vi "Main.vi"() -> ()   [LabVIEW 2021]
uses:
  Bronkhorst M13 Flow Meter/Settings Cluster.ctl
  Bronkhorst M13 Flow Meter/Bronkhorst M13 Flow Meter.lvlib
panel:
  in  "stop":bool
  in  "Bronkhorst Settings in":T1={"VISA resource name"="", "Simulated?"=FALSE, "Smoothing Steps"=1} {"Smoothing Steps" min=1 step=1}
  out "error out":errorcluster
  out "Flow Error":bool
  out "Temp Error":bool
  out "Setpoint Error":bool
  in  "Setpoint (%)":dbl
  out "Temp (C)":sgl
  out "flow":dbl
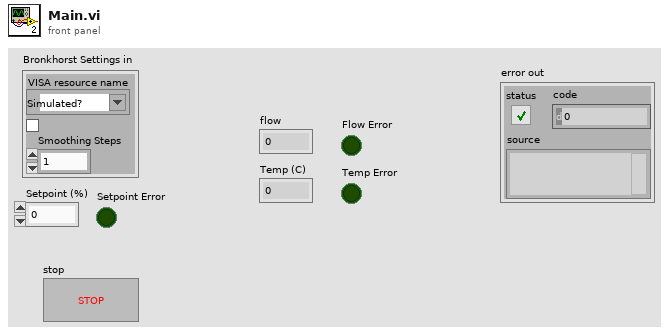
[diagram p1: front panel]
types:
  T1 = typedef "Bronkhorst M13 Flow Meter.lvlib/Settings Cluster.ctl" = cluster{"VISA resource name":refnum<visa-resource-name>, "Simulated?":bool, "Smoothing Steps":i32}
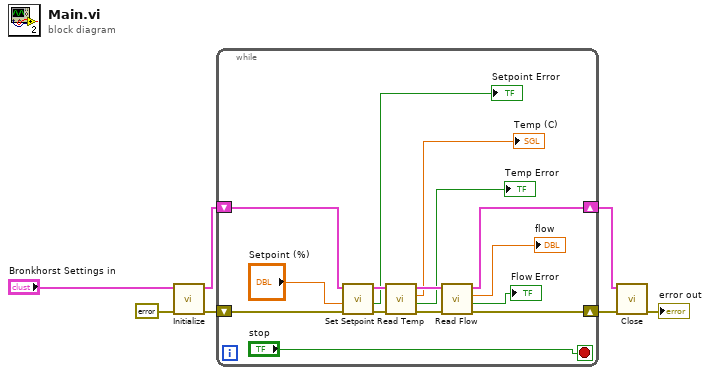
[diagram p0: block diagram]
diagram:
  n1 = call "Initialize.vi"("error in (no error)"=errorcluster {"status"=FALSE, "code"=0, "source"=""}, "Bronkhorst Settings in"="Bronkhorst Settings in") -> ("error out"=w6:errorcluster, "Bronkhorst Settings out"=w7:T1)  [unwired: 7 in, 1 out]
  n2 = while {
    shift-right: [w9] -> w5
    shift-left: w7 -> [w22]
    shift-right: [w8] -> w4
    shift-left: w6 -> [w21]
    stop <- "stop" stop-if-true
    n3 = call "Set Setpoint.vi"("error in (no error)"=w21, "Setpoint (%)"="Setpoint (%)", "Bronkhorst Settings in"=w22) -> ("error out"=w19:errorcluster, "Connection Error"=→"Setpoint Error":bool, "Bronkhorst Settings out"=w20:T1)  [unwired: 6 in]
    n4 = call "Read Temp.vi"("error in (no error)"=w19, "Bronkhorst Settings in"=w20) -> ("error out"=w17:errorcluster, "Connection Error"=→"Temp Error":bool, "Temp (C)"=→"Temp (C)":sgl, "Bronkhorst Settings out"=w18:T1)  [unwired: 6 in]
    n5 = call "Read Flow.vi"("error in (no error)"=w17, "Bronkhorst Settings in"=w18) -> ("error out"=w8:errorcluster, "Connection Error"=→"Flow Error":bool, "flow"=→"flow":dbl, "Bronkhorst Settings out"=w9:T1)  [unwired: 6 in]
  }
  n6 = call "Close.vi"("error in (no error)"=w4, "Bronkhorst Settings in"=w5) -> ("error out"=→"error out":errorcluster)  [unwired: 8 in, 1 out]
